vi "temperature_fpga.vi"() -> ()   [LabVIEW 2011]
uses:
  <vilib>/rvi/eio/common/nirviEmuTemplateMethod_errors.vi
  <vilib>/eio/EIONode/EIONode.xnode
panel:
  in  "Count(mSec)":u32=500
  out "error out":errorcluster
  out "Mod4/TC0":fxp<+/-,24,-2> format="%#_4g"
  out "Mod4/TC1":fxp<+/-,24,-2> format="%#_4g"
  out "Mod4/TC2":fxp<+/-,24,-2> format="%#_4g"
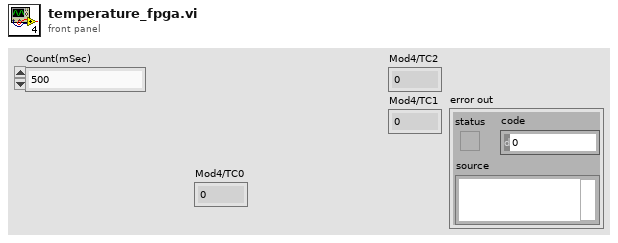
[diagram p1: front panel]
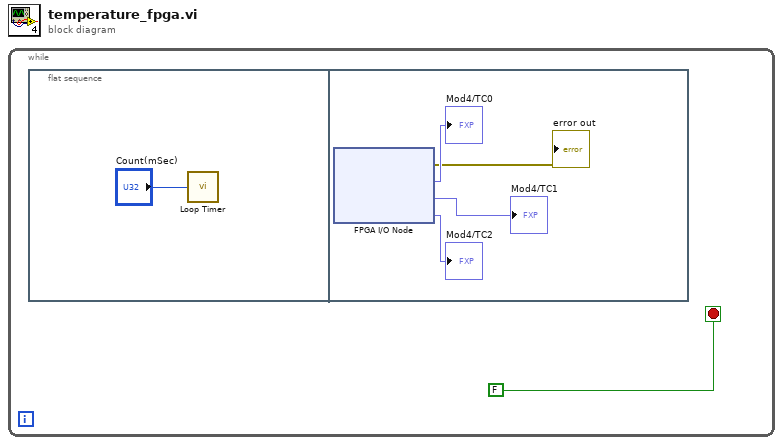
[diagram p0: block diagram]
diagram:
  n1 = while {
    stop <- FALSE ("stop") stop-if-true
    n2 = flat-sequence {
      frame #0 {
        n3 = call "Loop Timer"("Count(mSec)"="Count(mSec)") -> ()  [unwired: 1 out]
      }
      frame #1 {
        n4 = xnode "FPGA I/O Node"() -> ("error out"=→"error out":errorcluster, "Mod4/TC0"=→"Mod4/TC0":fxp<+/-,24,-2>, "Mod4/TC1"=→"Mod4/TC1":fxp<+/-,24,-2>, "Mod4/TC2"=→"Mod4/TC2":fxp<+/-,24,-2>)  [unwired: 4 in, 3 out]
      }
    }
  }
